vi "AddString.vi"(8 "error in (no error)":errorcluster, 10 "String":string, 11 "BreadcrumbNavigation in":refnum<class "BreadcrumbNavigator.lvclass">) -> (0 "error out":errorcluster, 3 "BreadcrumbNavigation out":refnum<class "BreadcrumbNavigator.lvclass">)   [LabVIEW 2015, in "BreadcrumbNavigator.lvclass"]
uses:
  BreadcrumbNavigator.lvclass
  BreadcrumbNavigator.lvclass/BreadcrumbNavigator.ctl
  Read Strings[].vi
  Write Strings[].vi
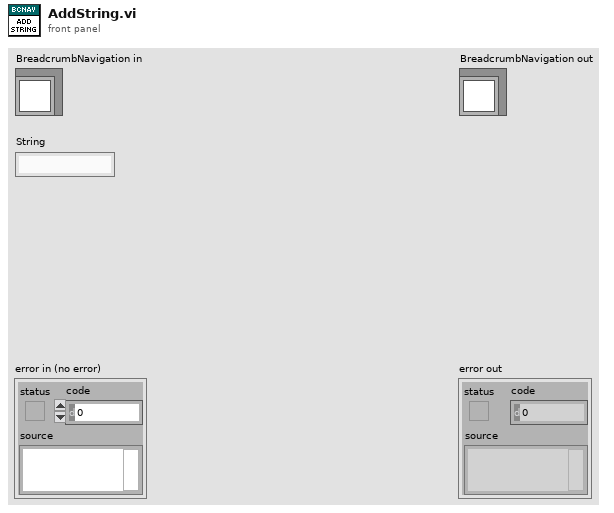
[diagram p1: front panel]
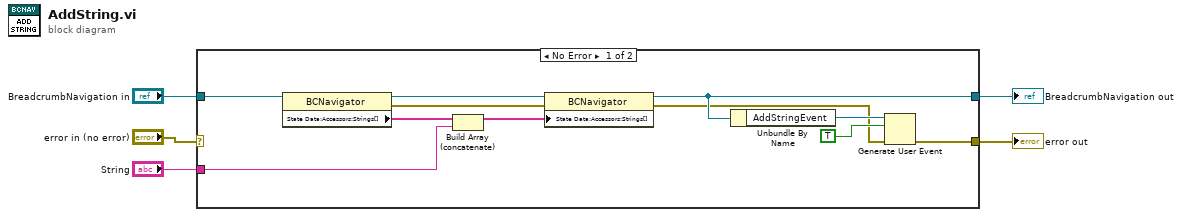
[diagram p0: block diagram]
diagram:
  n1 = case shown="No Error" "error in (no error)" {
    selector: "error in (no error)" -> [_ w18]
    tunnel: [w6 w18] -> w4
    tunnel: [w10 w17] -> w2
    tunnel: "BreadcrumbNavigation in" -> [w16 w17]
    tunnel: "String" -> [w12 _]
    frame No Error {
      n2 = property class="BCNavigator"(reference=w16) -> (reference out=w15:refnum<class "BreadcrumbNavigator.lvclass">, error out=w14:errorcluster, "State Data:Accessors:Strings[]"=w13:string[])  [unwired: 1 in]
      n3 = Build Array (concatenate)(w13, w12) -> (w11:string[])
      n4 = property class="BCNavigator"(reference=w15, error in=w14, "State Data:Accessors:Strings[]"=w11) -> (reference out=w10:refnum<class "BreadcrumbNavigator.lvclass">, error out=w7:errorcluster)
      n5 = Unbundle By Name(w10) -> ("AddStringEvent"=w9:refnum<user-event>)
      n6 = Generate User Event(user event=w9, event data cluster=TRUE, error in=w7) -> (error out=w6:errorcluster)  [unwired: 1 in, 1 out]
    }
    frame Error {
    }
  }
  "error out" <- w4
  "BreadcrumbNavigation out" <- w2
